vi "CF-data_filepath.vi"(11 "Input path":string) -> (2 "data Path + input":path, 3 "data Path":path)   [LabVIEW 2020, in "CF-common_features.lvlib"]
uses:
  CF-common_features.lvlib
panel:
  out "Common Path":path
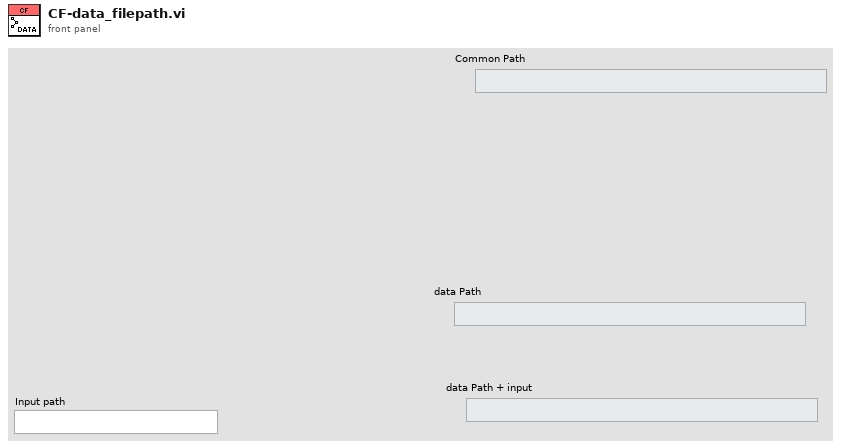
[diagram p1: front panel]
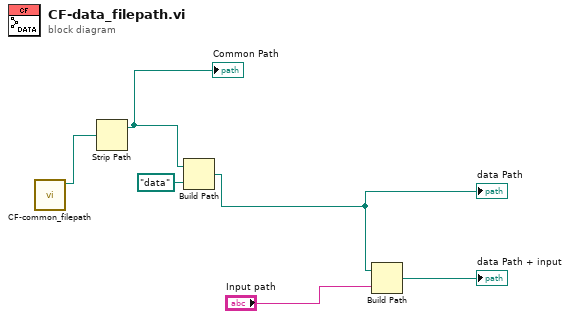
[diagram p0: block diagram]
diagram:
  n1 = call "CF-common_filepath.vi"() -> ("Common Path"=w4:path)  [unwired: 10 in, 1 out]
  n2 = Strip Path(path=w4) -> (stripped path=w3:path)  [unwired: 1 out]
  "Common Path" <- w3
  n3 = Build Path(base path=w3, name or relative path=path "data") -> (appended path=w1:path)
  "data Path" <- w1
  n4 = Build Path(base path=w1, name or relative path="Input path") -> (appended path=→"data Path + input":path)
